vi "ExtractArmpressure.vi"(11 "Arm pressure":T2(array[cluster])) -> (3 "output cluster":T1)   [LabVIEW 2013, in "main.lvlib"]
uses:
  main.lvlib
  <vilib>/GPower/String/GPString.lvlib
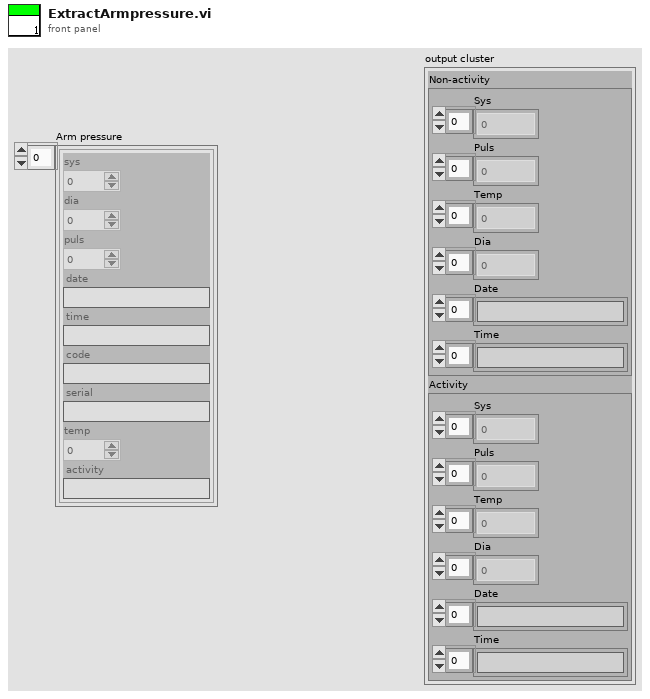
[diagram p1: front panel]
types:
  T1 = cluster{"Non-activity":cluster{"Sys":dbl[], "Dia":dbl[], "Puls":dbl[], "Temp":dbl[], "Date":string[], "Time":string[]}, "Activity":cluster{"Sys":dbl[], "Dia":dbl[], "Puls":dbl[], "Temp":dbl[], "Date":string[], "Time":string[]}}
  T2 = cluster{"sys":dbl, "dia":dbl, "puls":dbl, "date":string, "time":string, "code":string, "serial":string, "temp":dbl, "activity":string}[]
  T3 = cluster{"Sys":dbl[], "Dia":dbl[], "Puls":dbl[], "Temp":dbl[], "Date":string[], "Time":string[]}
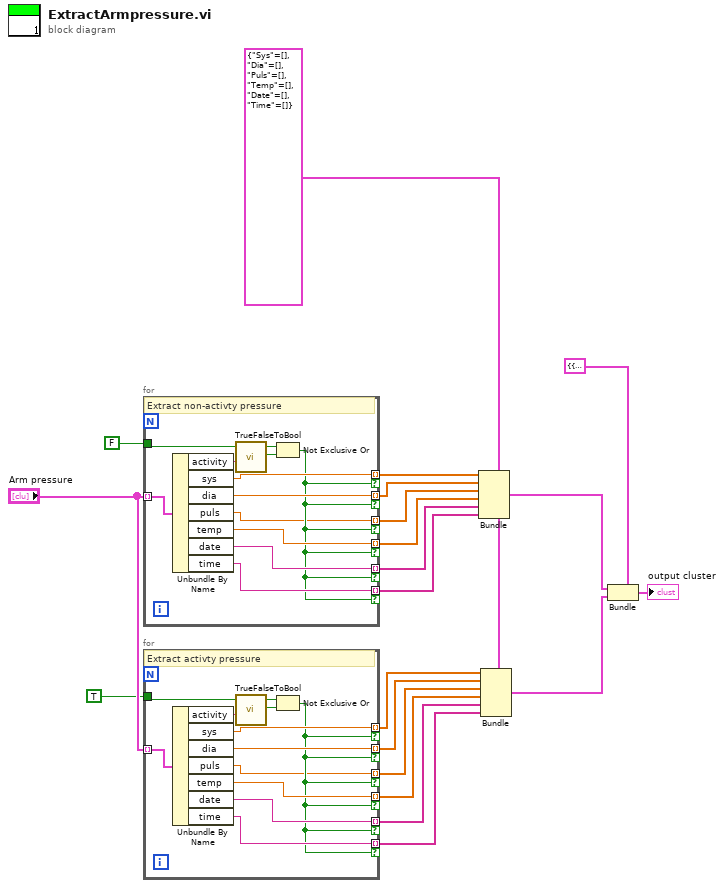
[diagram p0: block diagram]
diagram:
  w18 = T3 {"Sys"=[], "Dia"=[], "Puls"=[], "Temp"=[], "Date"=[], "Time"=[]}
  n1 = for {
    tunnel: "Arm pressure" -> [w31] mode=indexing
    tunnel: [w26] -> w17 mode=indexing if=w22
    tunnel: [w21] -> w15 mode=indexing if=w22
    tunnel: [w30] -> w14 mode=indexing if=w22
    tunnel: FALSE -> [w27]
    tunnel: [w25] -> w16 mode=indexing if=w22
    tunnel: [w24] -> w13 mode=indexing if=w22
    tunnel: [w23] -> w12 mode=indexing if=w22
    # "Extract non-activty pressure"
    n2 = Unbundle By Name(w31) -> ("activity"=w29:string, "sys"=w26:dbl, "dia"=w25:dbl, "puls"=w21:dbl, "temp"=w30:dbl, "date"=w24:string, "time"=w23:string)
    n3 = call <vilib>:"TrueFalseToBool.vi"("String"=w29) -> ("Boolean"=w28:bool)
    n4 = Not Exclusive Or(1:w28, 2:w27) -> (0:w22:bool)
  }
  n5 = for {
    tunnel: "Arm pressure" -> [w42] mode=indexing
    tunnel: [w37] -> w9 mode=indexing if=w33
    tunnel: [w32] -> w7 mode=indexing if=w33
    tunnel: [w41] -> w6 mode=indexing if=w33
    tunnel: TRUE -> [w38]
    tunnel: [w36] -> w8 mode=indexing if=w33
    tunnel: [w35] -> w5 mode=indexing if=w33
    tunnel: [w34] -> w4 mode=indexing if=w33
    # "Extract activty pressure"
    n6 = Unbundle By Name(w42) -> ("activity"=w40:string, "sys"=w37:dbl, "dia"=w36:dbl, "puls"=w32:dbl, "temp"=w41:dbl, "date"=w35:string, "time"=w34:string)
    n7 = call <vilib>:"TrueFalseToBool.vi"("String"=w40) -> ("Boolean"=w39:bool)
    n8 = Not Exclusive Or(1:w39, 2:w38) -> (0:w33:bool)
  }
  n9 = Bundle(cluster=w18, "Sys"=w17, "Dia"=w16, "Puls"=w15, "Temp"=w14, "Date"=w13, "Time"=w12) -> (w2:T3)
  n10 = Bundle(cluster=w18, "Sys"=w9, "Dia"=w8, "Puls"=w7, "Temp"=w6, "Date"=w5, "Time"=w4) -> (w3:T3)
  n11 = Bundle(cluster=T1 {"Non-activity"={"Sys"=[], "Dia"=[], "Puls"=[], "Temp"=[], "Date"=[], "Time"=[]}, "Activity"={"Sys"=[], "Dia"=[], "Puls"=[], "Temp"=[], "Date"=[], "Time"=[]}}, "Non-activity"=w2, "Activity"=w3) -> (→"output cluster":T1)
